vi "ReverseRandomArray.vi"() -> ()   [LabVIEW 2025]
panel:
  out "Reversed Array":dbl[](array[numeric])
  out "Array":dbl[](array[numeric])
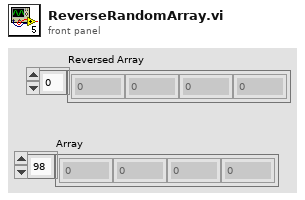
[diagram p1: front panel]
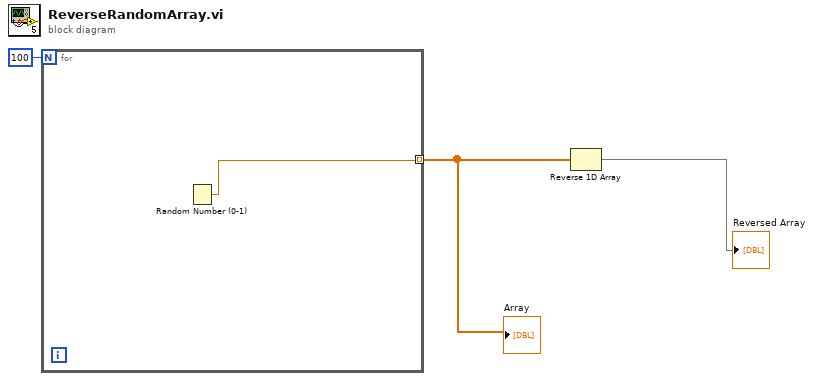
[diagram p0: block diagram]
diagram:
  n1 = for {
    N: 100 -> [_]
    tunnel: [w4] -> w2 mode=indexing
    n2 = Random Number (0-1)() -> (number: 0 to 1=w4:dbl)
  }
  "Array" <- w2
  n3 = Reverse 1D Array(array=w2) -> (reversed array=→"Reversed Array":dbl[])
